vi "Set MCM Calculation Settings.vi"(6 "Backend engine":T1, 8 "error in":errorcluster, 11 "MCM Calcualtion Settings":T2={"Repeats"=100, "Verbose"=TRUE, "Parallelization method"=enum."Single Core", "Processors"=1, "Temporary directory"=".", "Randomize"=TRUE} {"Processors" min=1 step=1; "Repeats" min=1 step=1}) -> (0 "error out":errorcluster)   [LabVIEW 2013, in "QWTBLVLib.lvlib"]
doc: "Set calculation settings for Monte Carlo method."
uses:
  QWTBLVLib.lvlib
  TD MCM Calculation Settings.ctl
  TD MCM Calculation Method.ctl
  TD Backend Engine.ctl
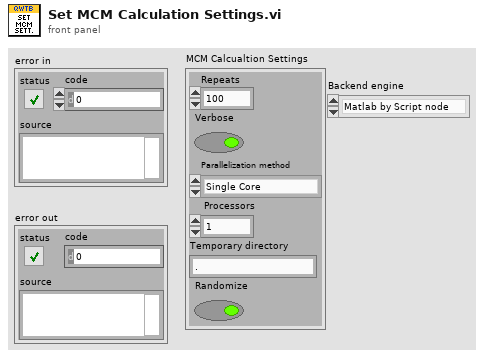
[diagram p1: front panel]
types:
  T1 = typedef "QWTBLVLib.lvlib/TD Backend Engine.ctl" = enum16{"Matlab by Script node", "GNU Octave by GOLPI"}
  T2 = typedef "QWTBLVLib.lvlib/TD MCM Calculation Settings.ctl" = cluster{"Repeats":i32, "Verbose":bool, "Parallelization method":T3, "Processors":i32, "Temporary directory":string, "Randomize":bool}
  T3 = typedef "QWTBLVLib.lvlib/TD MCM Calculation Method.ctl" = enum16{"Single Core", "Multi Core", "Multi Station"}
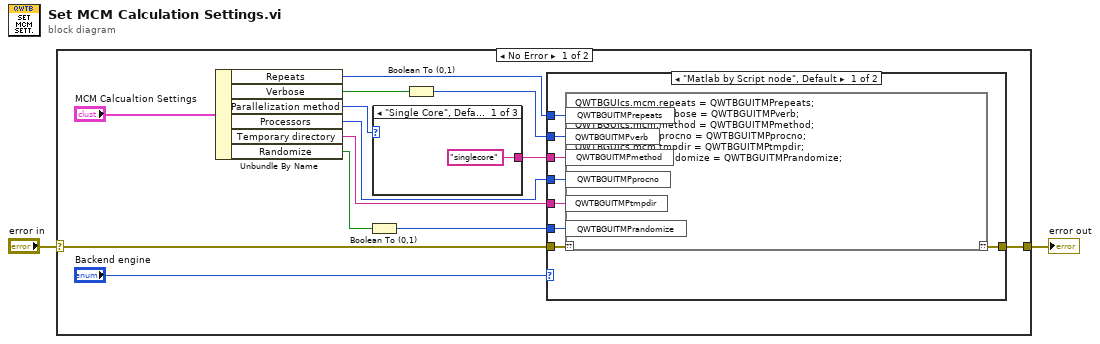
[diagram p0: block diagram]
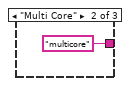
[diagram p3: hidden frame]
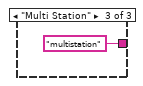
[diagram p4: hidden frame]
diagram:
  n1 = case shown="No Error" "error in" {
    selector: "error in" -> [w13 w28]
    tunnel: [w9 w28] -> w2
    frame No Error {
      n2 = Unbundle By Name("MCM Calcualtion Settings") -> ("Repeats"=w8:i32, "Verbose"=w12:bool, "Parallelization method"=w10:T3, "Processors"=w7:i32, "Temporary directory"=w6:string, "Randomize"=w5:bool)
      n3 = Boolean To (0,1)(Boolean=w5) -> (0, 1=w4:i16)
      n4 = case shown="\"Single Core\", Default" w10 {
        tunnel: ["singlecore" ("String") "multicore" ("String") "multistation" ("String")] -> w14
        frame "Single Core", Default {
        }
        frame "Multi Core" {
        }
        frame "Multi Station" {
        }
      }
      n5 = Boolean To (0,1)(Boolean=w12) -> (0, 1=w15:i16)
      n6 = case shown="\"Matlab by Script node\", Default" "Backend engine" {
        tunnel: [w23 w24] -> w9
        tunnel: w15 -> [w22 _]
        tunnel: w14 -> [w21 _]
        tunnel: w13 -> [w20 w24]
        tunnel: w8 -> [w19 _]
        tunnel: w7 -> [w18 _]
        tunnel: w6 -> [w17 _]
        tunnel: w4 -> [w16 _]
        frame "Matlab by Script node", Default {
          n7 = script code="QWTBGUIcs.mcm.repeats = QWTBGUITMPrepeats;\nQWTBGUIcs.mcm.verbose = QWTBGUITMPverb;\nQWTBGUIcs.mcm.method = QWTBGUITMPmethod;\nQWTBGUIcs.mcm.procno = QWTBGUITMPprocno;\nQWTBGUIcs.mcm.tmpdir = QWTBGUITMPtmpdir;\nQWTBGUIcs.mcm.randomize = QWTBGUITMPrandomize;"("??"=w20, "QWTBGUITMPverb"=w22, "QWTBGUITMPmethod"=w21, "QWTBGUITMPrepeats"=w19, "QWTBGUITMPprocno"=w18, "QWTBGUITMPtmpdir"=w17, "QWTBGUITMPrandomize"=w16) -> ("??"=w23:errorcluster)
        }
        frame "GNU Octave by GOLPI" {
          # "#2DO"
        }
      }
    }
    frame Error {
    }
  }
  "error out" <- w2
